vi "shutdown.vi"(8 "error in":errorcluster, 11 "websocket handler in":refnum<class "websocket upgrade handler.lvclass">) -> (0 "error out":errorcluster)   [LabVIEW 2016, in "websocket upgrade handler.lvclass"]
uses:
  websocket upgrade handler.lvclass
  websocket upgrade handler.lvclass/websocket upgrade handler.ctl
  user plugin/websocket user plugin.lvclass
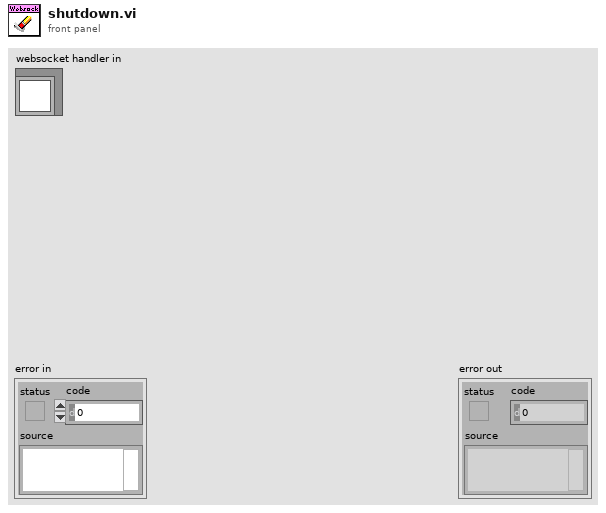
[diagram p1: front panel]
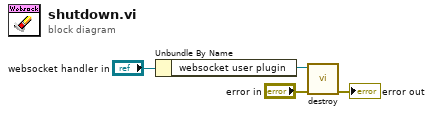
[diagram p0: block diagram]
diagram:
  n1 = Unbundle By Name("websocket handler in") -> ("websocket user plugin"=w1:refnum<class "websocket user plugin.lvclass">)
  n2 = call-dynamic "destroy.vi"("error in"="error in", "websocket user plugin in"=w1) -> ("error out"=→"error out":errorcluster)  [unwired: 9 in]
